vi "VerifPrevErrors.vi"(8 "error in (no error)":errorcluster, 11 "S4GUI in":refnum<class "S4GUI.lvclass">) -> (0 "error out":errorcluster, 3 "S4GUI out":refnum<class "S4GUI.lvclass">)   [LabVIEW 2018, in "S4GUI.lvclass"]
uses:
  S4GUI.lvclass
  Server/Server.lvclass/Server.ctl
  S4GUI.lvclass/S4GUI.ctl
  Acquisition/Acquisition.lvclass
  C:/Users/devstaff/sparc4/s4gui/Versao ZeroMQ REQ-REP/SPARC4_GUI -v1.0.9 - novo comportamento aba TEST/Server/Server.lvclass
  Channel/Channel.lvclass
  StateMachine/State Machine.lvclass
  Server/Server.lvclass
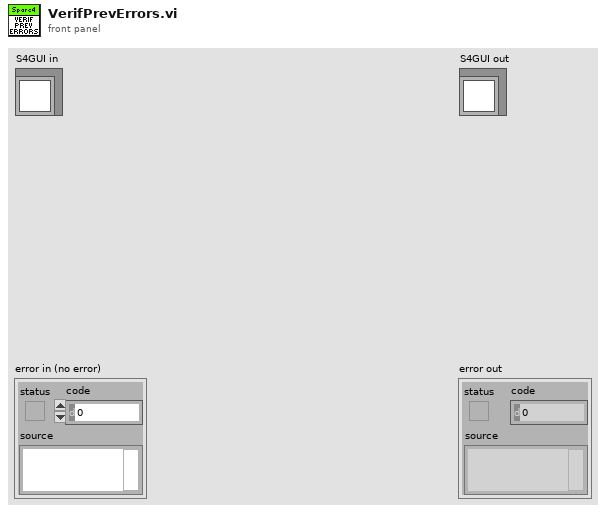
[diagram p1: front panel]
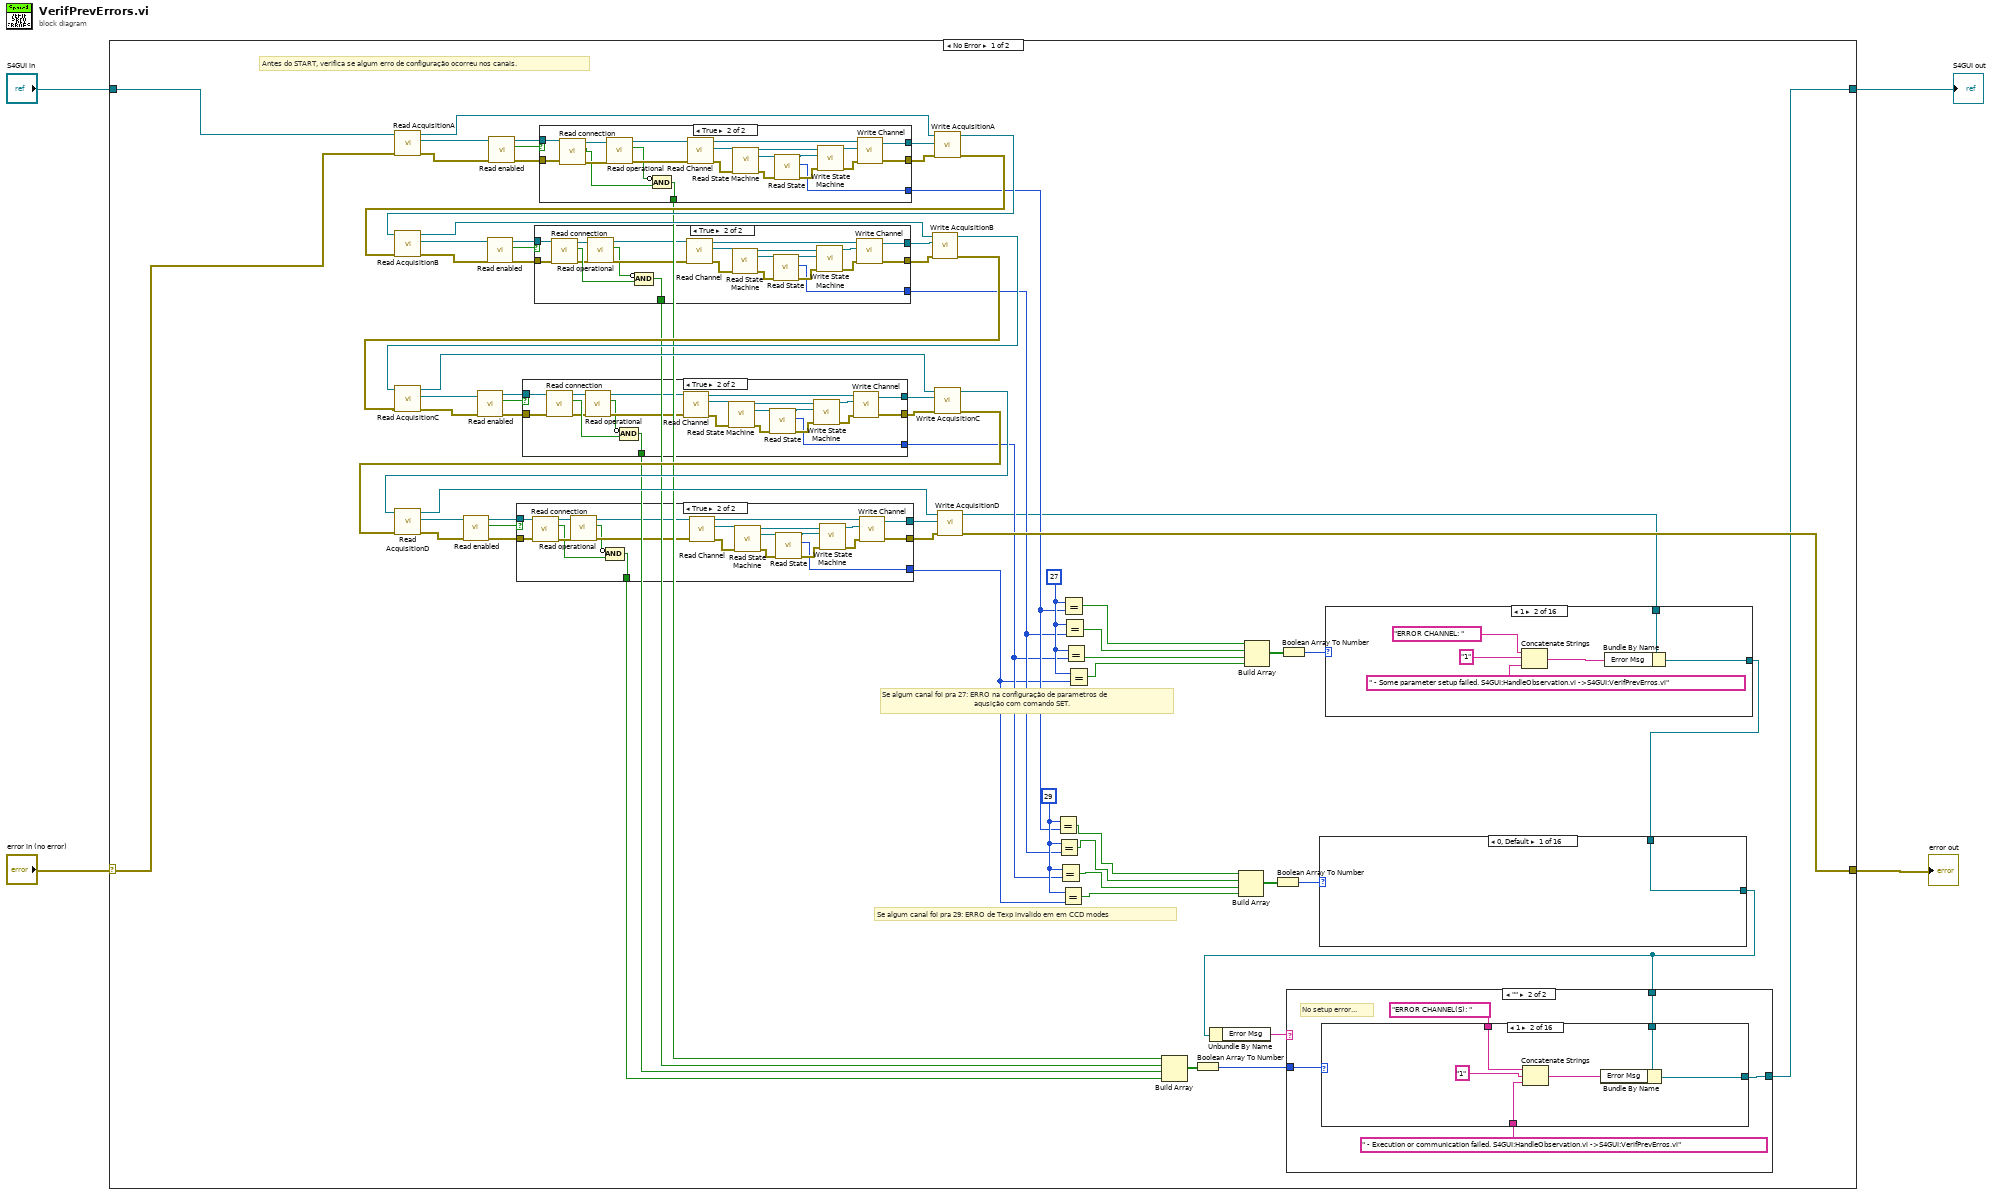
[diagram p0: block diagram]
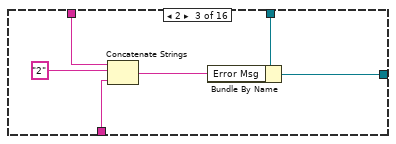
[diagram p4: hidden frame]
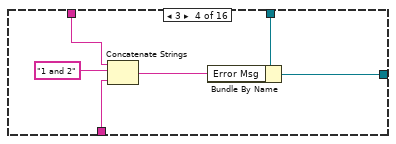
[diagram p5: hidden frame]
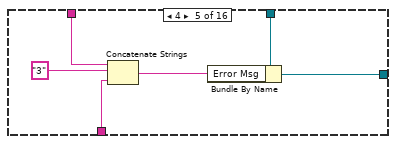
[diagram p6: hidden frame]
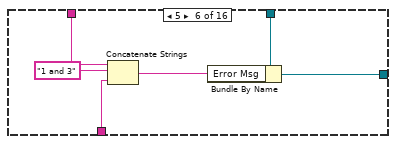
[diagram p7: hidden frame]
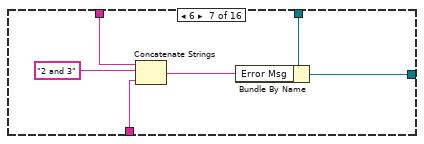
[diagram p8: hidden frame]
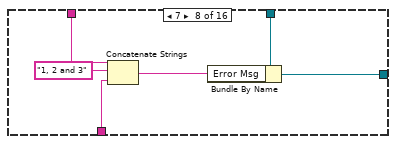
[diagram p9: hidden frame]
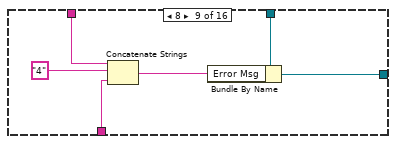
[diagram p10: hidden frame]
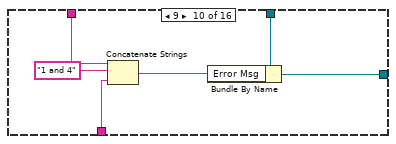
[diagram p11: hidden frame]
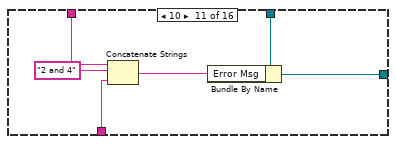
[diagram p12: hidden frame]
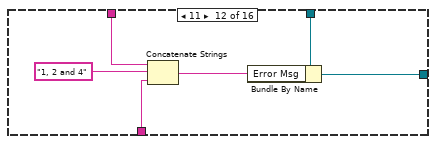
[diagram p13: hidden frame]
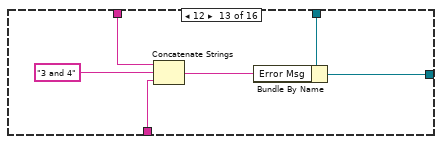
[diagram p14: hidden frame]
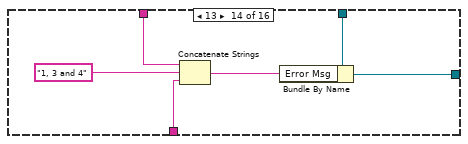
[diagram p15: hidden frame]
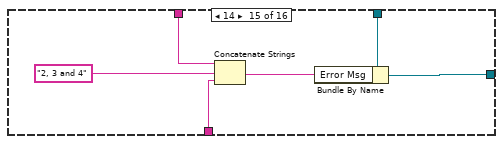
[diagram p16: hidden frame]
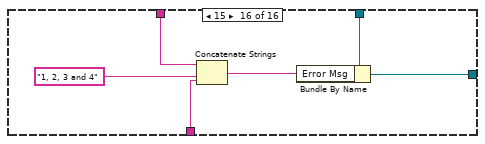
[diagram p17: hidden frame]
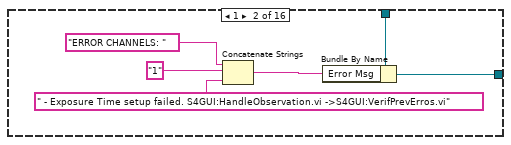
[diagram p18: hidden frame]
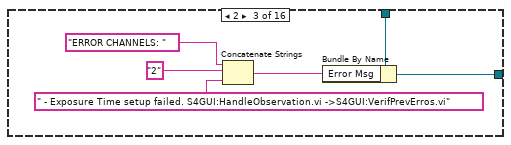
[diagram p19: hidden frame]
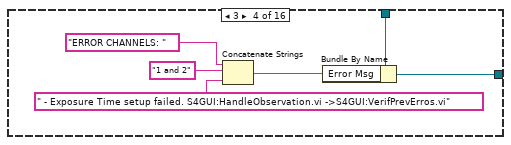
[diagram p20: hidden frame]
diagram:
  n1 = case shown="No Error" "error in (no error)" {
    selector: "error in (no error)" -> [w29 w461]
    tunnel: [w30 w461] -> w3
    tunnel: [w9 w460] -> w1
    tunnel: "S4GUI in" -> [w31 w460]
    frame No Error {
      w28 = 29 ("x")
      w36 = 27 ("x")
      # "Se algum canal foi pra 29: ERRO de Texp invalido em em CCD modes"
      # "Antes do START, verifica se algum erro de configuração ocorreu nos canais."
      # "Se algum canal foi pra 27: ERRO na configuração de parametros de\n                                              aqusição com comando SET."
      n2 = call-dynamic "Read AcquisitionA.vi"("error in (no error)"=w29, "S4ACS_GUI in"=w31) -> ("error out"=w62:errorcluster, "Acquisition.lvclass"=w63:refnum<class "Acquisition.lvclass">, "S4ACS_GUI out"=w73:refnum<class "S4GUI.lvclass">)  [unwired: 7 in]
      n3 = call-dynamic "Read enabled.vi"("error in (no error)"=w62, "Server in"=w63) -> ("error out"=w60:errorcluster, "enabled"=w59:bool, "Server out"=w61:refnum<class "Acquisition.lvclass">)  [unwired: 7 in]
      n4 = case shown="True" w59 {
        tunnel: w61 -> [w436 w444]
        tunnel: w60 -> [w435 w442]
        tunnel: [w436 w458] -> w74
        tunnel: [w435 w457] -> w72
        tunnel: [0 ("State") w447] -> w23
        tunnel: [FALSE ("operational") w438] -> w5
        frame False {
        }
        frame True {
          n5 = call "Read connection.vi"("error in (no error)"=w442, "Server in"=w444) -> ("error out"=w441:errorcluster, "connection"=w439:bool, "Server out"=w443:refnum<class "Acquisition.lvclass">)  [unwired: 7 in]
          n6 = call-dynamic "Read operational.vi"("error in (no error)"=w441, "Server in"=w443) -> ("error out"=w445:errorcluster, "operational"=w440:bool, "Server out"=w446:refnum<class "Acquisition.lvclass">)  [unwired: 7 in]
          n7 = Compound Arithmetic op=AND(invert w440, w439) -> (w438:bool)
          n8 = call-dynamic "Read Channel.vi"("error in (no error)"=w445, "Acquisition in"=w446) -> ("error out"=w456:errorcluster, "Channel.lvclass"=w455:refnum<class "Channel.lvclass">, "Acquisition out"=w459:refnum<class "Acquisition.lvclass">)  [unwired: 7 in]
          n9 = call-dynamic "Read State Machine.vi"("error in (no error)"=w456, "Device in"=w455) -> ("error out"=w449:errorcluster, "State Machine.lvclass"=w451:refnum<class "State Machine.lvclass">, "Device out"=w453:refnum<class "Channel.lvclass">)  [unwired: 7 in]
          n10 = call-dynamic "Read State.vi"("error in (no error)"=w449, "State Machine in"=w451) -> ("error out"=w448:errorcluster, "State"=w447:i32, "State Machine out"=w450:refnum<class "State Machine.lvclass">)  [unwired: 7 in]
          n11 = call-dynamic "Write State Machine.vi"("error in (no error)"=w448, "State Machine.lvclass"=w450, "Device in"=w453) -> ("error out"=w452:errorcluster, "Device out"=w454:refnum<class "Channel.lvclass">)  [unwired: 7 in]
          n12 = call-dynamic "Write Channel.vi"("error in (no error)"=w452, "Channel.lvclass"=w454, "Acquisition in"=w459) -> ("error out"=w457:errorcluster, "Acquisition out"=w458:refnum<class "Acquisition.lvclass">)  [unwired: 7 in]
        }
      }
      n13 = call-dynamic "Write AcquisitionA.vi"("error in (no error)"=w72, "Acquisition.lvclass"=w74, "S4ACS_GUI in"=w73) -> ("error out"=w69:errorcluster, "S4ACS_GUI out"=w68:refnum<class "S4GUI.lvclass">)  [unwired: 7 in]
      n14 = call "Read AcquisitionB.vi"("error in (no error)"=w69, "S4ACS_GUI in"=w68) -> ("error out"=w54:errorcluster, "Acquisition.lvclass"=w57:refnum<class "Acquisition.lvclass">, "S4ACS_GUI out"=w58:refnum<class "S4GUI.lvclass">)  [unwired: 7 in]
      n15 = call-dynamic "Read enabled.vi"("error in (no error)"=w54, "Server in"=w57) -> ("error out"=w53:errorcluster, "enabled"=w55:bool, "Server out"=w56:refnum<class "Acquisition.lvclass">)  [unwired: 7 in]
      n16 = case shown="True" w55 {
        tunnel: w56 -> [w410 w413]
        tunnel: w53 -> [w409 w415]
        tunnel: [w410 w432] -> w52
        tunnel: [w409 w431] -> w51
        tunnel: [0 ("State") w421] -> w22
        tunnel: [FALSE ("operational") w416] -> w8
        frame False {
        }
        frame True {
          n17 = call "Read connection.vi"("error in (no error)"=w415, "Server in"=w413) -> ("error out"=w414:errorcluster, "connection"=w418:bool, "Server out"=w412:refnum<class "Acquisition.lvclass">)  [unwired: 7 in]
          n18 = call-dynamic "Read operational.vi"("error in (no error)"=w414, "Server in"=w412) -> ("error out"=w419:errorcluster, "operational"=w417:bool, "Server out"=w420:refnum<class "Acquisition.lvclass">)  [unwired: 7 in]
          n19 = Compound Arithmetic op=AND(invert w417, w418) -> (w416:bool)
          n20 = call-dynamic "Read Channel.vi"("error in (no error)"=w419, "Acquisition in"=w420) -> ("error out"=w430:errorcluster, "Channel.lvclass"=w429:refnum<class "Channel.lvclass">, "Acquisition out"=w433:refnum<class "Acquisition.lvclass">)  [unwired: 7 in]
          n21 = call-dynamic "Read State Machine.vi"("error in (no error)"=w430, "Device in"=w429) -> ("error out"=w423:errorcluster, "State Machine.lvclass"=w425:refnum<class "State Machine.lvclass">, "Device out"=w427:refnum<class "Channel.lvclass">)  [unwired: 7 in]
          n22 = call-dynamic "Read State.vi"("error in (no error)"=w423, "State Machine in"=w425) -> ("error out"=w422:errorcluster, "State"=w421:i32, "State Machine out"=w424:refnum<class "State Machine.lvclass">)  [unwired: 7 in]
          n23 = call-dynamic "Write State Machine.vi"("error in (no error)"=w422, "State Machine.lvclass"=w424, "Device in"=w427) -> ("error out"=w426:errorcluster, "Device out"=w428:refnum<class "Channel.lvclass">)  [unwired: 7 in]
          n24 = call-dynamic "Write Channel.vi"("error in (no error)"=w426, "Channel.lvclass"=w428, "Acquisition in"=w433) -> ("error out"=w431:errorcluster, "Acquisition out"=w432:refnum<class "Acquisition.lvclass">)  [unwired: 7 in]
        }
      }
      n25 = call "Write AcquisitionB.vi"("error in (no error)"=w51, "Acquisition.lvclass"=w52, "S4ACS_GUI in"=w58) -> ("error out"=w67:errorcluster, "S4ACS_GUI out"=w66:refnum<class "S4GUI.lvclass">)  [unwired: 7 in]
      n26 = call-dynamic "Read AcquisitionC.vi"("error in (no error)"=w67, "S4ACS_GUI in"=w66) -> ("error out"=w49:errorcluster, "Acquisition.lvclass"=w50:refnum<class "Acquisition.lvclass">, "S4ACS_GUI out"=w71:refnum<class "S4GUI.lvclass">)  [unwired: 7 in]
      n27 = call-dynamic "Read enabled.vi"("error in (no error)"=w49, "Server in"=w50) -> ("error out"=w48:errorcluster, "enabled"=w46:bool, "Server out"=w47:refnum<class "Acquisition.lvclass">)  [unwired: 7 in]
      n28 = case shown="True" w46 {
        tunnel: w47 -> [w384 w389]
        tunnel: w48 -> [w383 w388]
        tunnel: [w384 w406] -> w45
        tunnel: [w383 w405] -> w44
        tunnel: [0 ("State") w395] -> w21
        tunnel: [FALSE ("operational") w390] -> w7
        frame False {
        }
        frame True {
          n29 = call "Read connection.vi"("error in (no error)"=w388, "Server in"=w389) -> ("error out"=w387:errorcluster, "connection"=w391:bool, "Server out"=w386:refnum<class "Acquisition.lvclass">)  [unwired: 7 in]
          n30 = call-dynamic "Read operational.vi"("error in (no error)"=w387, "Server in"=w386) -> ("error out"=w393:errorcluster, "operational"=w392:bool, "Server out"=w394:refnum<class "Acquisition.lvclass">)  [unwired: 7 in]
          n31 = Compound Arithmetic op=AND(invert w392, w391) -> (w390:bool)
          n32 = call-dynamic "Read Channel.vi"("error in (no error)"=w393, "Acquisition in"=w394) -> ("error out"=w404:errorcluster, "Channel.lvclass"=w403:refnum<class "Channel.lvclass">, "Acquisition out"=w407:refnum<class "Acquisition.lvclass">)  [unwired: 7 in]
          n33 = call-dynamic "Read State Machine.vi"("error in (no error)"=w404, "Device in"=w403) -> ("error out"=w397:errorcluster, "State Machine.lvclass"=w399:refnum<class "State Machine.lvclass">, "Device out"=w401:refnum<class "Channel.lvclass">)  [unwired: 7 in]
          n34 = call-dynamic "Read State.vi"("error in (no error)"=w397, "State Machine in"=w399) -> ("error out"=w396:errorcluster, "State"=w395:i32, "State Machine out"=w398:refnum<class "State Machine.lvclass">)  [unwired: 7 in]
          n35 = call-dynamic "Write State Machine.vi"("error in (no error)"=w396, "State Machine.lvclass"=w398, "Device in"=w401) -> ("error out"=w400:errorcluster, "Device out"=w402:refnum<class "Channel.lvclass">)  [unwired: 7 in]
          n36 = call-dynamic "Write Channel.vi"("error in (no error)"=w400, "Channel.lvclass"=w402, "Acquisition in"=w407) -> ("error out"=w405:errorcluster, "Acquisition out"=w406:refnum<class "Acquisition.lvclass">)  [unwired: 7 in]
        }
      }
      n37 = call-dynamic "Write AcquisitionC.vi"("error in (no error)"=w44, "Acquisition.lvclass"=w45, "S4ACS_GUI in"=w71) -> ("error out"=w65:errorcluster, "S4ACS_GUI out"=w64:refnum<class "S4GUI.lvclass">)  [unwired: 7 in]
      n38 = call-dynamic "Read AcquisitionD.vi"("error in (no error)"=w65, "S4ACS_GUI in"=w64) -> ("error out"=w41:errorcluster, "Acquisition.lvclass"=w43:refnum<class "Acquisition.lvclass">, "S4ACS_GUI out"=w70:refnum<class "S4GUI.lvclass">)  [unwired: 7 in]
      n39 = call-dynamic "Read enabled.vi"("error in (no error)"=w41, "Server in"=w43) -> ("error out"=w40:errorcluster, "enabled"=w39:bool, "Server out"=w42:refnum<class "Acquisition.lvclass">)  [unwired: 7 in]
      n40 = case shown="True" w39 {
        tunnel: w42 -> [w358 w366]
        tunnel: w40 -> [w357 w364]
        tunnel: [w358 w380] -> w38
        tunnel: [w357 w379] -> w37
        tunnel: [0 ("State") w369] -> w20
        tunnel: [FALSE ("operational") w360] -> w6
        frame False {
        }
        frame True {
          n41 = call "Read connection.vi"("error in (no error)"=w364, "Server in"=w366) -> ("error out"=w363:errorcluster, "connection"=w362:bool, "Server out"=w365:refnum<class "Acquisition.lvclass">)  [unwired: 7 in]
          n42 = call-dynamic "Read operational.vi"("error in (no error)"=w363, "Server in"=w365) -> ("error out"=w367:errorcluster, "operational"=w361:bool, "Server out"=w368:refnum<class "Acquisition.lvclass">)  [unwired: 7 in]
          n43 = Compound Arithmetic op=AND(invert w361, w362) -> (w360:bool)
          n44 = call-dynamic "Read Channel.vi"("error in (no error)"=w367, "Acquisition in"=w368) -> ("error out"=w378:errorcluster, "Channel.lvclass"=w377:refnum<class "Channel.lvclass">, "Acquisition out"=w381:refnum<class "Acquisition.lvclass">)  [unwired: 7 in]
          n45 = call-dynamic "Read State Machine.vi"("error in (no error)"=w378, "Device in"=w377) -> ("error out"=w371:errorcluster, "State Machine.lvclass"=w373:refnum<class "State Machine.lvclass">, "Device out"=w375:refnum<class "Channel.lvclass">)  [unwired: 7 in]
          n46 = call-dynamic "Read State.vi"("error in (no error)"=w371, "State Machine in"=w373) -> ("error out"=w370:errorcluster, "State"=w369:i32, "State Machine out"=w372:refnum<class "State Machine.lvclass">)  [unwired: 7 in]
          n47 = call-dynamic "Write State Machine.vi"("error in (no error)"=w370, "State Machine.lvclass"=w372, "Device in"=w375) -> ("error out"=w374:errorcluster, "Device out"=w376:refnum<class "Channel.lvclass">)  [unwired: 7 in]
          n48 = call-dynamic "Write Channel.vi"("error in (no error)"=w374, "Channel.lvclass"=w376, "Acquisition in"=w381) -> ("error out"=w379:errorcluster, "Acquisition out"=w380:refnum<class "Acquisition.lvclass">)  [unwired: 7 in]
        }
      }
      n49 = call-dynamic "Write AcquisitionD.vi"("error in (no error)"=w37, "Acquisition.lvclass"=w38, "S4ACS_GUI in"=w70) -> ("error out"=w30:errorcluster, "S4ACS_GUI out"=w17:refnum<class "S4GUI.lvclass">)  [unwired: 7 in]
      n50 = Equal?(x=w28, y=w23) -> (x = y?=w24:bool)
      n51 = Equal?(x=w28, y=w22) -> (x = y?=w25:bool)
      n52 = Equal?(x=w28, y=w21) -> (x = y?=w26:bool)
      n53 = Equal?(x=w28, y=w20) -> (x = y?=w27:bool)
      n54 = Equal?(x=w36, y=w23) -> (x = y?=w32:bool)
      n55 = Equal?(x=w36, y=w22) -> (x = y?=w33:bool)
      n56 = Equal?(x=w36, y=w21) -> (x = y?=w34:bool)
      n57 = Equal?(x=w36, y=w20) -> (x = y?=w35:bool)
      n58 = Build Array(w5, w8, w7, w6) -> (w13:bool[])
      n59 = Boolean Array To Number(Boolean array=w13) -> (number=w12:u32)
      n60 = Build Array(w24, w25, w26, w27) -> (w16:bool[])
      n61 = Build Array(w32, w33, w34, w35) -> (w19:bool[])
      n62 = Boolean Array To Number(Boolean array=w16) -> (number=w15:u32)
      n63 = Boolean Array To Number(Boolean array=w19) -> (number=w18:u32)
      n64 = case shown="1" w18 {
        tunnel: [w265 w266 w273 w278 w284 w290 w296 w302 w308 w314 w320 w326 w332 w338 w344 w350] -> w14
        tunnel: w17 -> [w264 w267 w272 w279 w285 w291 w297 w303 w309 w315 w321 w327 w333 w339 w345 w351]
        frame 0, Default {
          n65 = Bundle By Name(cluster=w264, "Error Msg"="") -> (w265:refnum<class "S4GUI.lvclass">)
        }
        frame 1 {
          n66 = Concatenate Strings("ERROR CHANNEL: ", "1", " - Some parameter setup failed. S4GUI:HandleObservation.vi ->S4GUI:VerifPrevErros.vi") -> (w271:string)
          n67 = Bundle By Name(cluster=w267, "Error Msg"=w271) -> (w266:refnum<class "S4GUI.lvclass">)
        }
        frame 2 {
          n68 = Concatenate Strings("ERROR CHANNEL: ", "2", " - Some parameter setup failed. S4GUI:HandleObservation.vi ->S4GUI:VerifPrevErros.vi") -> (w277:string)
          n69 = Bundle By Name(cluster=w272, "Error Msg"=w277) -> (w273:refnum<class "S4GUI.lvclass">)
        }
        frame 3 {
          n70 = Concatenate Strings("ERROR CHANNELS: ", "1 and 2", " - Some parameter setup failed. S4GUI:HandleObservation.vi ->S4GUI:VerifPrevErros.vi") -> (w283:string)
          n71 = Bundle By Name(cluster=w279, "Error Msg"=w283) -> (w278:refnum<class "S4GUI.lvclass">)
        }
        frame 4 {
          n72 = Concatenate Strings("ERROR CHANNEL: ", "3", " - Some parameter setup failed. S4GUI:HandleObservation.vi ->S4GUI:VerifPrevErros.vi") -> (w289:string)
          n73 = Bundle By Name(cluster=w285, "Error Msg"=w289) -> (w284:refnum<class "S4GUI.lvclass">)
        }
        frame 5 {
          n74 = Concatenate Strings("ERROR CHANNELS: ", "1 and 3", " -  Some parameter setup failed. S4GUI:HandleObservation.vi ->S4GUI:VerifPrevErros.vi") -> (w295:string)
          n75 = Bundle By Name(cluster=w291, "Error Msg"=w295) -> (w290:refnum<class "S4GUI.lvclass">)
        }
        frame 6 {
          n76 = Concatenate Strings("ERROR CHANNELS: ", "2 and 3", " - Some parameter setup failed. S4GUI:HandleObservation.vi ->S4GUI:VerifPrevErros.vi") -> (w301:string)
          n77 = Bundle By Name(cluster=w297, "Error Msg"=w301) -> (w296:refnum<class "S4GUI.lvclass">)
        }
        frame 7 {
          n78 = Concatenate Strings("ERROR CHANNELS: ", "1, 2 and 3", " -  Some parameter setup failed. S4GUI:HandleObservation.vi ->S4GUI:VerifPrevErros.vi") -> (w307:string)
          n79 = Bundle By Name(cluster=w303, "Error Msg"=w307) -> (w302:refnum<class "S4GUI.lvclass">)
        }
        frame 8 {
          n80 = Concatenate Strings("ERROR CHANNEL: ", "4", " - Some parameter setup failed. S4GUI:HandleObservation.vi ->S4GUI:VerifPrevErros.vi") -> (w313:string)
          n81 = Bundle By Name(cluster=w309, "Error Msg"=w313) -> (w308:refnum<class "S4GUI.lvclass">)
        }
        frame 9 {
          n82 = Concatenate Strings("ERROR CHANNELS: ", "1 and 4", " - Some parameter setup failed. S4GUI:HandleObservation.vi ->S4GUI:VerifPrevErros.vi") -> (w319:string)
          n83 = Bundle By Name(cluster=w315, "Error Msg"=w319) -> (w314:refnum<class "S4GUI.lvclass">)
        }
        frame 10 {
          n84 = Concatenate Strings("ERROR CHANNELS: ", "2 and 4", " - Some parameter setup failed. S4GUI:HandleObservation.vi ->S4GUI:VerifPrevErros.vi") -> (w325:string)
          n85 = Bundle By Name(cluster=w321, "Error Msg"=w325) -> (w320:refnum<class "S4GUI.lvclass">)
        }
        frame 11 {
          n86 = Concatenate Strings("ERROR CHANNELS: ", "1, 2 and 4", " - Some parameter setup failed. S4GUI:HandleObservation.vi ->S4GUI:VerifPrevErros.vi") -> (w331:string)
          n87 = Bundle By Name(cluster=w327, "Error Msg"=w331) -> (w326:refnum<class "S4GUI.lvclass">)
        }
        frame 12 {
          n88 = Concatenate Strings("ERROR CHANNELS: ", "3 and 4", "- Some parameter setup failed. S4GUI:HandleObservation.vi ->S4GUI:VerifPrevErros.vi") -> (w337:string)
          n89 = Bundle By Name(cluster=w333, "Error Msg"=w337) -> (w332:refnum<class "S4GUI.lvclass">)
        }
        frame 13 {
          n90 = Concatenate Strings("ERROR CHANNELS: ", "1, 3 and 4", " - Some parameter setup failed. S4GUI:HandleObservation.vi ->S4GUI:VerifPrevErros.vi") -> (w343:string)
          n91 = Bundle By Name(cluster=w339, "Error Msg"=w343) -> (w338:refnum<class "S4GUI.lvclass">)
        }
        frame 14 {
          n92 = Concatenate Strings("ERROR CHANNELS: ", "2, 3 and 4", " - Some parameter setup failed. S4GUI:HandleObservation.vi ->S4GUI:VerifPrevErros.vi") -> (w349:string)
          n93 = Bundle By Name(cluster=w345, "Error Msg"=w349) -> (w344:refnum<class "S4GUI.lvclass">)
        }
        frame 15 {
          n94 = Concatenate Strings("ERROR CHANNELS: ", "1, 2, 3 and 4", " -  Some parameter setup failed. S4GUI:HandleObservation.vi ->S4GUI:VerifPrevErros.vi") -> (w355:string)
          n95 = Bundle By Name(cluster=w351, "Error Msg"=w355) -> (w350:refnum<class "S4GUI.lvclass">)
        }
      }
      n96 = case shown="0, Default" w15 {
        tunnel: [w172 w173 w180 w185 w191 w197 w203 w209 w215 w221 w227 w233 w239 w245 w251 w257] -> w10
        tunnel: w14 -> [w172 w174 w179 w186 w192 w198 w204 w210 w216 w222 w228 w234 w240 w246 w252 w258]
        frame 0, Default {
        }
        frame 1 {
          n97 = Concatenate Strings("ERROR CHANNELS: ", "1", " - Exposure Time setup failed. S4GUI:HandleObservation.vi ->S4GUI:VerifPrevErros.vi") -> (w178:string)
          n98 = Bundle By Name(cluster=w174, "Error Msg"=w178) -> (w173:refnum<class "S4GUI.lvclass">)
        }
        frame 2 {
          n99 = Concatenate Strings("ERROR CHANNELS: ", "2", " - Exposure Time setup failed. S4GUI:HandleObservation.vi ->S4GUI:VerifPrevErros.vi") -> (w184:string)
          n100 = Bundle By Name(cluster=w179, "Error Msg"=w184) -> (w180:refnum<class "S4GUI.lvclass">)
        }
        frame 3 {
          n101 = Concatenate Strings("ERROR CHANNELS: ", "1 and 2", " - Exposure Time setup failed. S4GUI:HandleObservation.vi ->S4GUI:VerifPrevErros.vi") -> (w190:string)
          n102 = Bundle By Name(cluster=w186, "Error Msg"=w190) -> (w185:refnum<class "S4GUI.lvclass">)
        }
        frame 4 {
          n103 = Concatenate Strings("ERROR CHANNELS: ", "3", " - Exposure Time setup failed. S4GUI:HandleObservation.vi ->S4GUI:VerifPrevErros.vi") -> (w196:string)
          n104 = Bundle By Name(cluster=w192, "Error Msg"=w196) -> (w191:refnum<class "S4GUI.lvclass">)
        }
        frame 5 {
          n105 = Concatenate Strings("ERROR CHANNELS: ", "1 and 3", " - Exposure Time setup failed. S4GUI:HandleObservation.vi ->S4GUI:VerifPrevErros.vi") -> (w202:string)
          n106 = Bundle By Name(cluster=w198, "Error Msg"=w202) -> (w197:refnum<class "S4GUI.lvclass">)
        }
        frame 6 {
          n107 = Concatenate Strings("ERROR CHANNELS: ", "2 and 3", " - Exposure Time setup failed. S4GUI:HandleObservation.vi ->S4GUI:VerifPrevErros.vi") -> (w208:string)
          n108 = Bundle By Name(cluster=w204, "Error Msg"=w208) -> (w203:refnum<class "S4GUI.lvclass">)
        }
        frame 7 {
          n109 = Concatenate Strings("ERROR CHANNELS: ", "1, 2 and 3", " - Exposure Time setup failed. S4GUI:HandleObservation.vi ->S4GUI:VerifPrevErros.vi") -> (w214:string)
          n110 = Bundle By Name(cluster=w210, "Error Msg"=w214) -> (w209:refnum<class "S4GUI.lvclass">)
        }
        frame 8 {
          n111 = Concatenate Strings("ERROR CHANNELS: ", "4", " - Exposure Time setup failed. S4GUI:HandleObservation.vi ->S4GUI:VerifPrevErros.vi") -> (w220:string)
          n112 = Bundle By Name(cluster=w216, "Error Msg"=w220) -> (w215:refnum<class "S4GUI.lvclass">)
        }
        frame 9 {
          n113 = Concatenate Strings("ERROR CHANNELS: ", "1 and 4", " - Exposure Time setup failed. S4GUI:HandleObservation.vi ->S4GUI:VerifPrevErros.vi") -> (w226:string)
          n114 = Bundle By Name(cluster=w222, "Error Msg"=w226) -> (w221:refnum<class "S4GUI.lvclass">)
        }
        frame 10 {
          n115 = Concatenate Strings("ERROR CHANNELS: ", "2 and 4", " - Exposure Time setup failed. S4GUI:HandleObservation.vi ->S4GUI:VerifPrevErros.vi") -> (w232:string)
          n116 = Bundle By Name(cluster=w228, "Error Msg"=w232) -> (w227:refnum<class "S4GUI.lvclass">)
        }
        frame 11 {
          n117 = Concatenate Strings("ERROR CHANNELS: ", "1, 2 and 4", " - Exposure Time setup failed. S4GUI:HandleObservation.vi ->S4GUI:VerifPrevErros.vi") -> (w238:string)
          n118 = Bundle By Name(cluster=w234, "Error Msg"=w238) -> (w233:refnum<class "S4GUI.lvclass">)
        }
        frame 12 {
          n119 = Concatenate Strings("ERROR CHANNELS: ", "3 and 4", " - Exposure Time setup failed. S4GUI:HandleObservation.vi ->S4GUI:VerifPrevErros.vi") -> (w244:string)
          n120 = Bundle By Name(cluster=w240, "Error Msg"=w244) -> (w239:refnum<class "S4GUI.lvclass">)
        }
        frame 13 {
          n121 = Concatenate Strings("ERROR CHANNELS: ", "1, 3 and 4", " - Exposure Time setup failed. S4GUI:HandleObservation.vi ->S4GUI:VerifPrevErros.vi") -> (w250:string)
          n122 = Bundle By Name(cluster=w246, "Error Msg"=w250) -> (w245:refnum<class "S4GUI.lvclass">)
        }
        frame 14 {
          n123 = Concatenate Strings("ERROR CHANNELS: ", "2, 3 and 4", " - Exposure Time setup failed. S4GUI:HandleObservation.vi ->S4GUI:VerifPrevErros.vi") -> (w256:string)
          n124 = Bundle By Name(cluster=w252, "Error Msg"=w256) -> (w251:refnum<class "S4GUI.lvclass">)
        }
        frame 15 {
          n125 = Concatenate Strings("ERROR CHANNELS: ", "1, 2, 3 and 4", " - Exposure Time setup failed. S4GUI:HandleObservation.vi ->S4GUI:VerifPrevErros.vi") -> (w262:string)
          n126 = Bundle By Name(cluster=w258, "Error Msg"=w262) -> (w257:refnum<class "S4GUI.lvclass">)
        }
      }
      n127 = Unbundle By Name(w10) -> ("Error Msg"=w11:string)
      n128 = case shown="\"\"" w11 {
        tunnel: w12 -> [_ w80]
        tunnel: w10 -> [w75 w79]
        tunnel: [w75 w78] -> w9
        frame Default {
          # "Some setup error already occurred."
        }
        frame "" {
          # "No setup error..."
          n129 = case shown="1" w80 {
            tunnel: [w81 w84 w91 w96 w102 w108 w114 w120 w126 w132 w138 w144 w150 w156 w162 w168] -> w78
            tunnel: w79 -> [w81 w85 w90 w97 w103 w109 w115 w121 w127 w133 w139 w145 w151 w157 w163 w169]
            tunnel: "ERROR CHANNEL(S): " -> [_ w83 w89 w95 w101 w107 w113 w119 w125 w131 w137 w143 w149 w155 w161 w167]
            tunnel: " - Execution or communication failed. S4GUI:HandleObservation.vi ->S4GUI:VerifPrevErros.vi" -> [_ w82 w88 w94 w100 w106 w112 w118 w124 w130 w136 w142 w148 w154 w160 w166]
            frame 0, Default {
            }
            frame 1 {
              n130 = Concatenate Strings(w83, "1", w82) -> (w87:string)
              n131 = Bundle By Name(cluster=w85, "Error Msg"=w87) -> (w84:refnum<class "S4GUI.lvclass">)
            }
            frame 2 {
              n132 = Concatenate Strings(w89, "2", w88) -> (w93:string)
              n133 = Bundle By Name(cluster=w90, "Error Msg"=w93) -> (w91:refnum<class "S4GUI.lvclass">)
            }
            frame 3 {
              n134 = Concatenate Strings(w95, "1 and 2", w94) -> (w99:string)
              n135 = Bundle By Name(cluster=w97, "Error Msg"=w99) -> (w96:refnum<class "S4GUI.lvclass">)
            }
            frame 4 {
              n136 = Concatenate Strings(w101, "3", w100) -> (w105:string)
              n137 = Bundle By Name(cluster=w103, "Error Msg"=w105) -> (w102:refnum<class "S4GUI.lvclass">)
            }
            frame 5 {
              n138 = Concatenate Strings(w107, "1 and 3", w106) -> (w111:string)
              n139 = Bundle By Name(cluster=w109, "Error Msg"=w111) -> (w108:refnum<class "S4GUI.lvclass">)
            }
            frame 6 {
              n140 = Concatenate Strings(w113, "2 and 3", w112) -> (w117:string)
              n141 = Bundle By Name(cluster=w115, "Error Msg"=w117) -> (w114:refnum<class "S4GUI.lvclass">)
            }
            frame 7 {
              n142 = Concatenate Strings(w119, "1, 2 and 3", w118) -> (w123:string)
              n143 = Bundle By Name(cluster=w121, "Error Msg"=w123) -> (w120:refnum<class "S4GUI.lvclass">)
            }
            frame 8 {
              n144 = Concatenate Strings(w125, "4", w124) -> (w129:string)
              n145 = Bundle By Name(cluster=w127, "Error Msg"=w129) -> (w126:refnum<class "S4GUI.lvclass">)
            }
            frame 9 {
              n146 = Concatenate Strings(w131, "1 and 4", w130) -> (w135:string)
              n147 = Bundle By Name(cluster=w133, "Error Msg"=w135) -> (w132:refnum<class "S4GUI.lvclass">)
            }
            frame 10 {
              n148 = Concatenate Strings(w137, "2 and 4", w136) -> (w141:string)
              n149 = Bundle By Name(cluster=w139, "Error Msg"=w141) -> (w138:refnum<class "S4GUI.lvclass">)
            }
            frame 11 {
              n150 = Concatenate Strings(w143, "1, 2 and 4", w142) -> (w147:string)
              n151 = Bundle By Name(cluster=w145, "Error Msg"=w147) -> (w144:refnum<class "S4GUI.lvclass">)
            }
            frame 12 {
              n152 = Concatenate Strings(w149, "3 and 4", w148) -> (w153:string)
              n153 = Bundle By Name(cluster=w151, "Error Msg"=w153) -> (w150:refnum<class "S4GUI.lvclass">)
            }
            frame 13 {
              n154 = Concatenate Strings(w155, "1, 3 and 4", w154) -> (w159:string)
              n155 = Bundle By Name(cluster=w157, "Error Msg"=w159) -> (w156:refnum<class "S4GUI.lvclass">)
            }
            frame 14 {
              n156 = Concatenate Strings(w161, "2, 3 and 4", w160) -> (w165:string)
              n157 = Bundle By Name(cluster=w163, "Error Msg"=w165) -> (w162:refnum<class "S4GUI.lvclass">)
            }
            frame 15 {
              n158 = Concatenate Strings(w167, "1, 2, 3 and 4", w166) -> (w171:string)
              n159 = Bundle By Name(cluster=w169, "Error Msg"=w171) -> (w168:refnum<class "S4GUI.lvclass">)
            }
          }
        }
      }
    }
    frame Error {
    }
  }
  "error out" <- w3
  "S4GUI out" <- w1
